vi "Drive Encoder Z Filter.vi"   [LabVIEW 2009]
uses:
  Motor Control Global.vi
  <vilib>/rvi/FXPMathLib/FxpSub/XNode/nifxpmath_Sub.xnode
  <vilib>/rvi/FXPMathLib/FxpSub/subVIs/nifxpmath_Sub_SimConfig.ctl
  <vilib>/fxp/LVFixedPointQuantizationPolicyTypeDef.ctl
  <vilib>/fxp/LVFixedPointOverflowPolicyTypeDef.ctl
  <vilib>/rvi/FXPMathLib/FxpSub/simVIs/DllFxpSubTemp_sub.vi
  <vilib>/rvi/FXPMathLib/FxpAdd/XNode/nifxpmath_Add.xnode
  <vilib>/rvi/FXPMathLib/FxpAdd/subVIs/nifxpmath_Add_SimConfig.ctl
  <vilib>/rvi/FXPMathLib/FxpAdd/simVIs/DllFxpAddTemp_sub.vi
  <vilib>/rvi/FXPMathLib/FxpMul/XNode/nifxpmath_Multiplier.xnode
  <vilib>/rvi/FXPMathLib/FxpMul/subVIs/nifxpmath_Mul_SimConfig.ctl
  <vilib>/rvi/FXPMathLib/FxpMul/simVIs/DllFxpMulTemp_sub.vi
  <vilib>/rvi/Analysis/measure/butterworth/XNode/niFpgaButterworthFilter.xnode
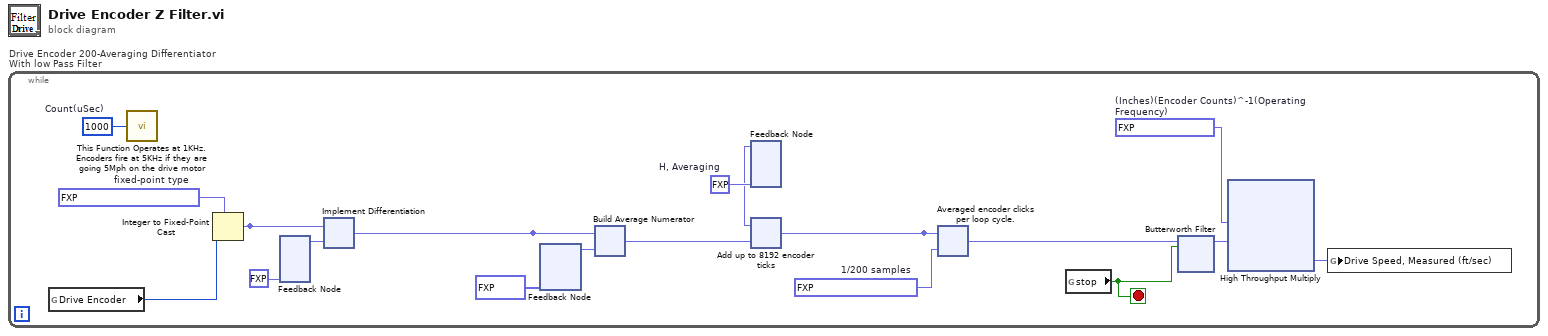
[diagram p0: block diagram]
diagram:
  n1 = while "Drive Encoder 200-Averaging Differentiator With low Pass Filter" {
    stop <- w5 stop-if-true
    w4 = fxp<+,18,3> 4.33551025390625  # (Inches)(Encoder Counts)^-1(Operating Frequency)
    w8 = fxp<+,11,-7> 0.005001068115234375  # 1/200 samples
    w13 = u32 1000  # Count(uSec)
    w11 = fxp<+/-,10,10> 0.0  # H, Averaging
    w18 = fxp<+/-,32,32> 0.0  # fixed-point type
    n2 = global read "Motor Control Global.vi" "Drive Encoder"() -> (w1:i32)
    n3 = call "This Function Operates at 1KHz. Encoders fire at 5KHz if they are going 5Mph on the drive motor"("Count(uSec)"=w13) -> ()  [unwired: 1 out]
    n4 = Integer to Fixed-Point Cast(fixed-point type=w18, integer=w1) -> (fixed-point=w17:fxp<+/-,32,32>)
    n5 = feedback #1(fxp<+/-,32,32> 0.0) -> (w16:fxp<+/-,32,32>)
    n6 = xnode "Implement Differentiation"("x"=w17, "y"=w16) -> ("x-y"=w14:fxp<+/-,4,4>)
    n7 = feedback #2(fxp<+/-,3,3>[] [0.0, 0.0, 0.0, 0.0, 0.0, 0.0, 0.0, 0.0, 0.0, 0.0, 0.0, 0.0, 0.0, 0.0, 0.0, 0.0, 0.0, 0.0, 0.0, 0.0, 0.0, 0.0, 0.0, 0.0, 0.0, 0.0, 0.0, 0.0, 0.0, 0.0, 0.0, 0.0, 0.0, 0.0, 0.0, 0.0, 0.0, 0.0, 0.0, 0.0, 0.0, 0.0, 0.0, 0.0, 0.0, 0.0, 0.0, 0.0, 0.0, 0.0, 0.0, 0.0, 0.0, 0.0, 0.0, 0.0, 0.0, 0.0, 0.0, 0.0, 0.0, 0.0, 0.0, 0.0, 0.0, 0.0, 0.0, 0.0, 0.0, 0.0, 0.0, 0.0, 0.0, 0.0, 0.0, 0.0, 0.0, 0.0, 0.0, 0.0, 0.0, 0.0, 0.0, 0.0, 0.0, 0.0, 0.0, 0.0, 0.0, 0.0, 0.0, 0.0, 0.0, 0.0, 0.0, 0.0, 0.0, 0.0, 0.0, 0.0, 0.0, 0.0, 0.0, 0.0, 0.0, 0.0, 0.0, 0.0, 0.0, 0.0, 0.0, 0.0, 0.0, 0.0, 0.0, 0.0, 0.0, 0.0, 0.0, 0.0, 0.0, 0.0, 0.0, 0.0, 0.0, 0.0, 0.0, 0.0, 0.0, 0.0, 0.0, 0.0, 0.0, 0.0, 0.0, 0.0, 0.0, 0.0, 0.0, 0.0, 0.0, 0.0, 0.0, 0.0, 0.0, 0.0, 0.0, 0.0, 0.0, 0.0, 0.0, 0.0, 0.0, 0.0, 0.0, 0.0, 0.0, 0.0, 0.0, 0.0, 0.0, 0.0, 0.0, 0.0, 0.0, 0.0, 0.0, 0.0, 0.0, 0.0, 0.0, 0.0, 0.0, 0.0, 0.0, 0.0, 0.0, 0.0, 0.0, 0.0, 0.0, 0.0, 0.0, 0.0, 0.0, 0.0, 0.0, 0.0, 0.0, 0.0, 0.0, 0.0, 0.0, 0.0, 0.0, 0.0, 0.0, 0.0, 0.0, 0.0]) -> (w15:fxp<+/-,4,4>)
    n8 = xnode "Build Average Numerator"("x"=w14, "y"=w15) -> ("x-y"=w10:fxp<+/-,5,5>)
    n9 = feedback #3(w11) -> (w9:fxp<+/-,13,13>)
    n10 = xnode "Add up to 8192 encoder ticks"("x"=w9, "y"=w10) -> ("x+y"=w7:fxp<+/-,13,13>)
    n11 = xnode "Averaged encoder clicks per loop cycle."("x"=w7, "y"=w8) -> ("x*y"=w6:fxp<+/-,18,6>)
    n12 = global read "Motor Control Global.vi" "stop"() -> (w5:bool)
    n13 = xnode "Butterworth Filter"("input data"=w6, "reset"=w5) -> ("output data"=w3:fxp<+/-,22,10>)  [unwired: 1 in]
    n14 = xnode "High Throughput Multiply"("x"=w4, "y"=w3) -> ("x*y"=w2:fxp<+/-,14,4>)
    n15 = global write "Motor Control Global.vi" "Drive Speed, Measured (ft/sec)"(w2) -> ()
  }
